vi "Numbers to match.vi"() -> ()   [LabVIEW 2015]
panel:
  out "# of iterations":dbl format="%#.0f"
  out "Current Number":dbl format="%#.0f"
  in  "Numbers to Match":dbl min=0.0 max=10000.0 step=1.0 format="%#.0f"
  # "*numeric indicator*"
  # "* numeric control*"
  # "Precision = 0"
  # "Default = 50"
  # "Min = 0 (coerce)"
  # "Max = 10000 (coerce)"
  # "Inc = 1 (coerce to nearest)"
  # "Precision = 0"
  # "*numeric indicator*"
  # "Precision = 0"
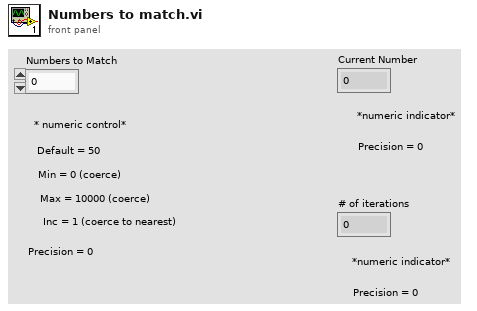
[diagram p1: front panel]
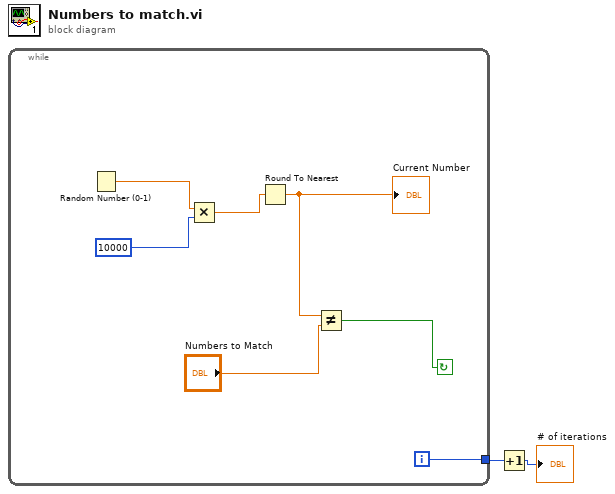
[diagram p0: block diagram]
diagram:
  n1 = while {
    tunnel: [w3] -> w1
    i -> [w3]
    stop <- w4 continue-if-true
    n2 = Random Number (0-1)() -> (number: 0 to 1=w6:dbl)
    n3 = Multiply(x=w6, y=10000) -> (x*y=w8:dbl)
    n4 = Round To Nearest(number=w8) -> (nearest integer value=w7:dbl)
    "Current Number" <- w7
    n5 = Not Equal?(x=w7, y="Numbers to Match") -> (x != y?=w4:bool)
  }
  n6 = Increment(x=w1) -> (x+1=→"# of iterations":i32)
